vi "cal_visa_out_pos.vi"(10 "Visa In Position":cluster{"Left":u32, "Top":i32}, 11 "Main Node Position":cluster{"Left":u32, "Top":i32}) -> (3 "Visa Out  Position":cluster{"Left":u32, "Top":i32})   [LabVIEW 2018]
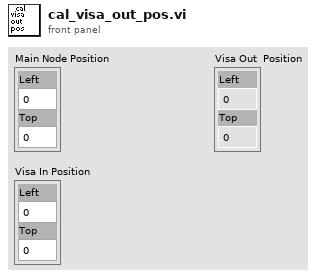
[diagram p1: front panel]
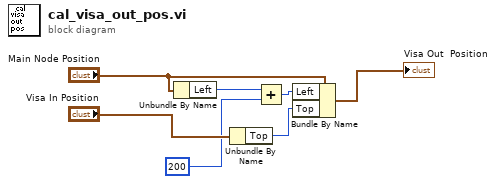
[diagram p0: block diagram]
diagram:
  n1 = Unbundle By Name("Main Node Position") -> ("Left"=w4:u32)
  n2 = Unbundle By Name("Visa In Position") -> ("Top"=w2:i32)
  n3 = Add(x=w4, y=u32 200 ("X Offset")) -> (x+y=w5:u32)
  n4 = Bundle By Name(cluster="Main Node Position", "Left"=w5, "Top"=w2) -> (→"Visa Out  Position":cluster{"Left":u32, "Top":i32})
